vi "smart_get.vi"(2 "Input Image":T3, 3 "Cluster":T2) -> (0 "Image Out":T3, 1 "Acquired Buffer Number":i32)   [LabVIEW 2010]
uses:
  <vilib>/vision/Image Controls.llb/IMAQ Image.ctl
  <vilib>/userDefined/High Color/IMAQdx.ctl
  <vilib>/vision/driver/NI_Vision_Acquisition_Software.lvlib
  <vilib>/vision/NI_Vision_Development_Module.lvlib
  Image-Stack-Compressor/Stack Reader Wrapper/labview vis/StackReaderWrapper.lvlib
panel:
  # "edited by MHG 10/20 to get frames from MMF"
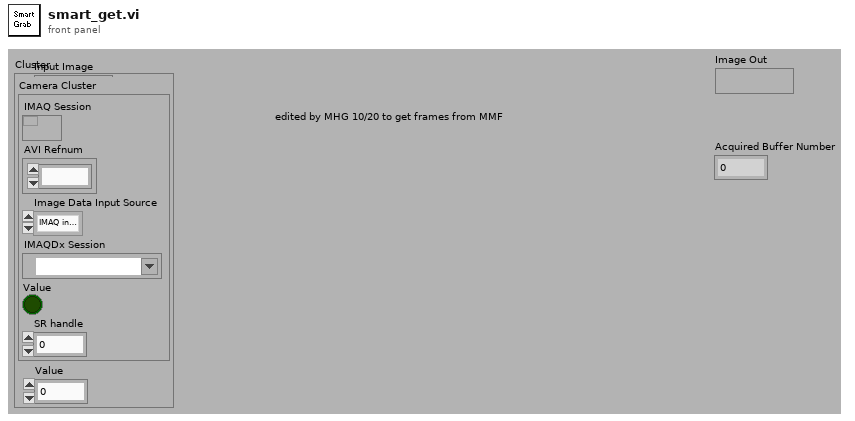
[diagram p1: front panel]
types:
  T1 = typedef "IMAQdx.ctl" = refnum<k21>
  T2 = cluster{"Camera Cluster":cluster{"IMAQ Session":refnum<k11>, "AVI Refnum":refnum<k1>, "Image Data Input Source":enum32{"IMAQ interface", "IMAQdx interface", "AVI file", "MMF File"}, "IMAQDx Session":T1, "Value":bool, "SR handle":u32}, "Value":i32}
  T3 = typedef "IMAQ Image.ctl" = refnum<image>
  T4 = typedef "Image Type" = u32
  T5 = cluster{"IMAQ Session":refnum<k11>, "AVI Refnum":refnum<k1>, "Image Data Input Source":enum32{"IMAQ interface", "IMAQdx interface", "AVI file", "MMF File"}, "IMAQDx Session":T1, "Value":bool, "SR handle":u32}
  T6 = enum32{"IMAQ interface", "IMAQdx interface", "AVI file", "MMF File"}
  T7 = typedef "AviRefnum.ctl" = refnum<k1>
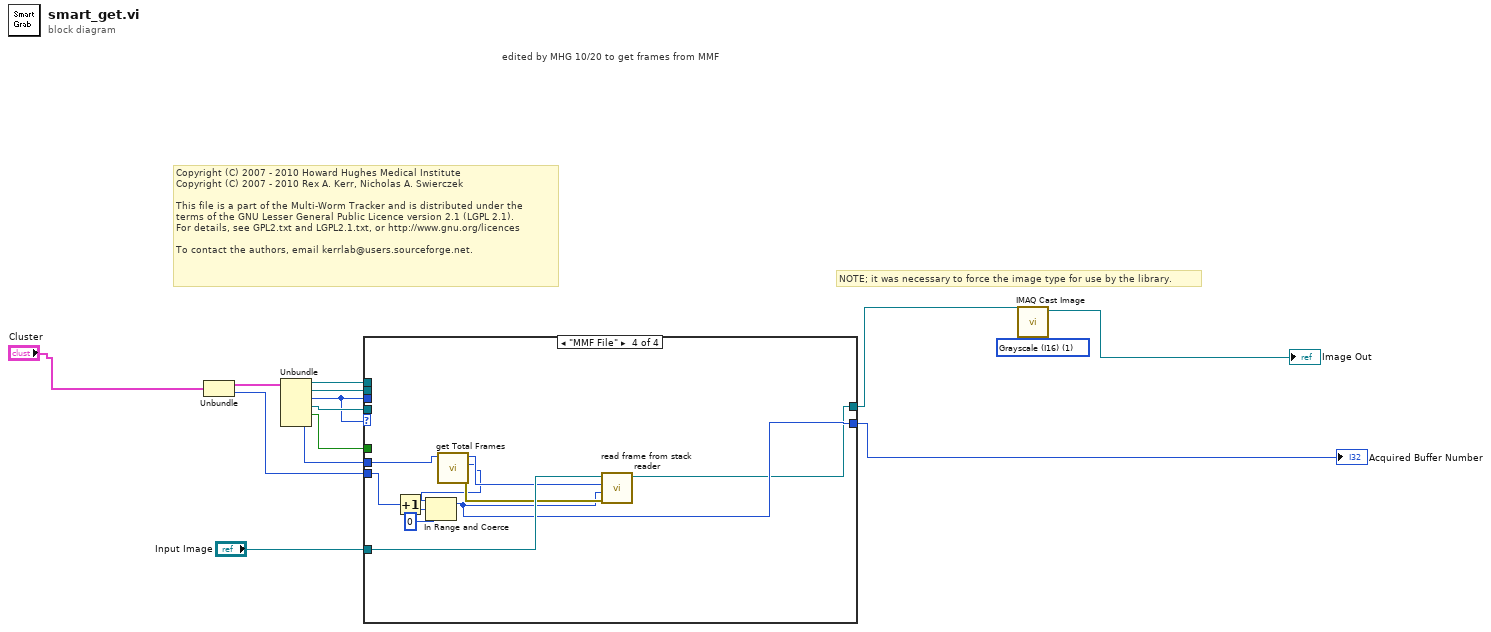
[diagram p0: block diagram]
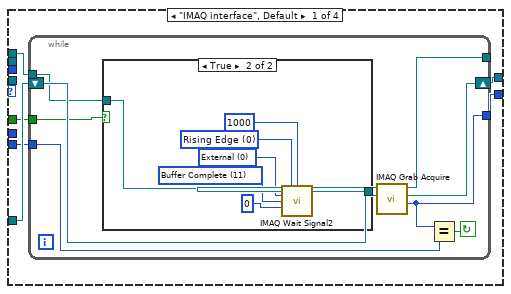
[diagram p2: hidden frame]
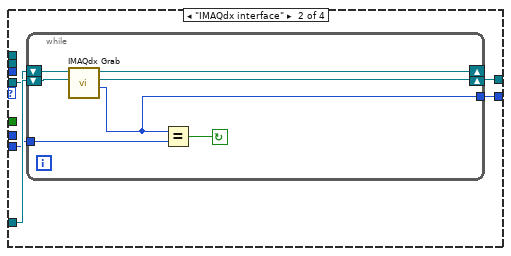
[diagram p4: hidden frame]
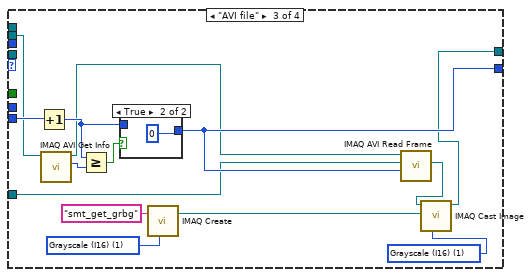
[diagram p5: hidden frame]
diagram:
  w5 = T4 1 items=["Grayscale (U8)", "Grayscale (I16)", "Grayscale (SGL)", "Complex (CSG)", "RGB (U32)", "HSL (U32)", "RGB (U64)"] ("Image Type")
  # "edited by MHG 10/20 to get frames from MMF"
  # "NOTE; it was necessary to force the image type for use by the library."
  # "Copyright (C) 2007 - 2010 Howard Hughes Medical Institute\nCopyright (C) 2007 - 2010 Rex A. Kerr, Nicholas A. Swierczek\n \nThis file is a part of the Multi-Worm Tracker and is distributed under the\nterms of the GNU Lesser General Public Licence version 2.1 (LGPL 2.1).\nFor details, see GPL2.txt and LGPL2.1.txt, or http://www.gnu.org/licences\n \nTo contact the authors, email kerrlab@users.sourceforge.net."
  n1 = Unbundle("Cluster") -> ("Camera Cluster"=w8:T5, "Value"=w12:i32)
  n2 = Unbundle(w8) -> ("IMAQ Session"=w14:refnum<k11>, "AVI Refnum"=w6:refnum<k1>, "Image Data Input Source"=w4:T6, "IMAQDx Session"=w7:T1, "Value"=w2:bool, "SR handle"=w1:u32)
  n3 = case shown="\"MMF File\"" w4 {
    tunnel: w7 -> [_ w40 _ _]
    tunnel: w14 -> [w20 _ _ _]
    tunnel: "Input Image" -> [w19 w42 w57 w75]
    tunnel: w12 -> [w18 w41 w63 w68]
    tunnel: [w17 w39 w55 w66] -> w9
    tunnel: [w16 w38 w59 w67] -> w11
    tunnel: w4 -> [_ _ _ _]
    tunnel: w6 -> [_ _ w50 _]
    tunnel: w2 -> [w15 _ _ _]
    tunnel: w1 -> [_ _ _ w73]
    frame "IMAQ interface", Default {
      n4 = while {
        tunnel: [w27] -> _
        tunnel: [w26] -> w16
        tunnel: w20 -> [w23]
        tunnel: w18 -> [w24]
        shift-right: [w28] -> w17
        shift-left: w19 -> [w25]
        tunnel: w15 -> [w21]
        stop <- w29 continue-if-true
        n5 = case shown="True" w21 {
          tunnel: w23 -> [w30 w36]
          tunnel: [w30 w37] -> w22
          frame False {
          }
          frame True {
            w32 = u32 0 items=["Rising Edge", "Falling Edge"] ("Signal polarity")
            w33 = u32 0 items=["External", "RTSI ", "ISO In", "ISO Out", "Status"] ("Signal Type")
            w34 = u32 11 items=["Acquisition in progress"=15, "Acquisition done"=8, "Frame start"=9, "Frame done"=10, "Buffer Complete"=11] ("Status Signal")
            n6 = call <vilib>:"IMAQ Wait Signal2.vi"("IMAQ Session In"=w36, "Signal polarity"=w32, "Timeout (ms)"=u32 1000, "Signal Type"=w33, "Status Signal"=w34, "Signal Number"=u32 0) -> ("IMAQ Session Out"=w37:refnum<k11>)  [unwired: 8 in, 1 out]
          }
        }
        n7 = call <vilib>:"IMAQ Grab Acquire.vi"("Image In"=w25, "IMAQ Session In"=w22) -> ("Acquired Buffer Number"=w26:u32, "Image Out"=w28:T3, "IMAQ Session Out"=w27:refnum<k11>)  [unwired: 6 in, 1 out]
        n8 = Equal?(x=w26, y=w24) -> (x = y?=w29:bool)
      }
    }
    frame "IMAQdx interface" {
      n9 = while {
        tunnel: [w46] -> w38
        tunnel: w41 -> [w43]
        shift-right: [w48] -> w39
        shift-left: w42 -> [w44]
        shift-right: [w47] -> _
        shift-left: w40 -> [w45]
        stop <- w49 continue-if-true
        n10 = call <vilib>:"IMAQdx Grab.vi"("Image In"=w44, "Session In"=w45) -> ("Buffer Number Out"=w46:u32, "Image Out"=w48:T3, "Session Out"=w47:T1)  [unwired: 6 in, 1 out]
        n11 = Equal?(x=w46, y=w43) -> (x = y?=w49:bool)
      }
    }
    frame "AVI file" {
      w53 = T4 1 items=["Grayscale (U8)", "Grayscale (I16)", "Grayscale (SGL)", "Complex (CSG)", "RGB (U32)", "HSL (U32)", "RGB (U64)"] ("Image Type")
      w54 = T4 1 items=["Grayscale (U8)", "Grayscale (I16)", "Grayscale (SGL)", "Complex (CSG)", "RGB (U32)", "HSL (U32)", "RGB (U64)"] ("Image Type")
      n12 = Increment(x=w63) -> (x+1=w61:i32)
      n13 = call "IMAQ AVI Get Info"("Avi Refnum"=w50) -> ("Number of Frames"=w62:u32, "Avi Refnum (duplicate)"=w58:T7)  [unwired: 6 in, 3 out]
      n14 = Greater Or Equal?(x=w61, y=w62) -> (x >= y?=w60:bool)
      n15 = case shown="True" w60 {
        tunnel: w61 -> [w64 _]
        tunnel: [w64 0] -> w59
        frame False {
        }
        frame True {
        }
      }
      n16 = call "IMAQ Create"("Image Name"="smt_get_grbg", "Image Type"=w53) -> ("New Image"=w51:T3)  [unwired: 3 in, 1 out]
      n17 = call "IMAQ AVI Read Frame"("Frame Number"=w59, "Image"=w57, "Avi Refnum"=w58) -> ("Image Out"=w56:T3)  [unwired: 5 in, 3 out]
      n18 = call "IMAQ Cast Image"("Image Type"=w54, "Image Dst"=w51, "Image Src"=w56) -> ("Image Dst Out"=w55:T3)  [unwired: 7 in, 1 out]
    }
    frame "MMF File" {
      n19 = Increment(x=w68) -> (x+1=w74:i32)
      n20 = call "get Total Frames.vi"("sr"=w73) -> ("error out"=w71:errorcluster, "function return"=w70:i32, "sr out"=w72:u32)  [unwired: 8 in]
      n21 = In Range and Coerce(upper limit=w70, x=w74, lower limit=0) -> (coerced(x)=w67:i32)  [unwired: 1 out]
      n22 = call "read frame from stack reader.vi"("error in (no error)"=w71, "frameNumber"=w67, "sr"=w72, "image dst"=w75) -> ("Image Out"=w66:T3)  [unwired: 6 in, 1 out]
    }
  }
  "Acquired Buffer Number" <- w11
  n23 = call "IMAQ Cast Image"("Image Type"=w5, "Image Src"=w9) -> ("Image Dst Out"=→"Image Out":T3)  [unwired: 8 in, 1 out]
